vi "tsapp_enable_bus_statistics.vi"(8 "错误输入（无错误）":errorcluster, 11 "Enable":bool) -> (0 "错误输出":errorcluster, 3 "tsapp_enable_bus_statistics":i32)   [LabVIEW 2016]
uses:
  TSMaster.dll
panel:
  # "功能：\n使能总线的数据统计功能，使能包含例如：标准帧/扩展帧的收发数量、总线负载率等信息统计"
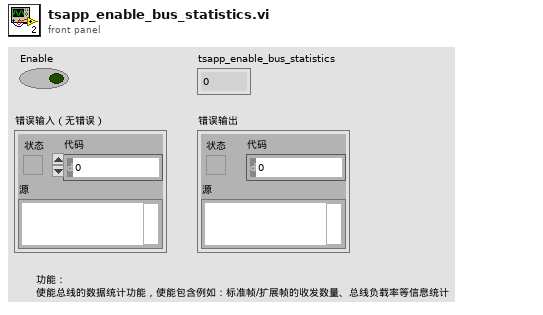
[diagram p1: front panel]
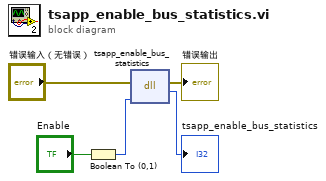
[diagram p0: block diagram]
diagram:
  n1 = Boolean To (0,1)(Boolean="Enable") -> (0, 1=w5:i16)
  n2 = dll-call lib="C:/Users/Eric/Desktop/LabVIEW/TSMasterAPI/Win32/TSMaster_LV2010_Release/TSMaster.dll" fn="tsapp_enable_bus_statistics"(error in="错误输入（无错误）", "AEnable"=w5) -> (error out=→"错误输出":errorcluster, "tsapp_enable_bus_statistics"=→"tsapp_enable_bus_statistics":i32)  [unwired: 3 in, 1 out]
